vi "LIN speichern.vi"(8 "error in (no error)":errorcluster caption="Fehler (Eingang, kein Fehler)", 10 "File Name LIN":T2, 11 "Pfad LIN":T1) -> (0 "error out":errorcluster, 2 ".LIN Datei Pfad":path, 3 "Pfad LIN out":T1)   [LabVIEW 2020, in "Linearisierung v2.lvlib"]
uses:
  Linearisierung v2.lvlib
  Visualisierungs Elemente/Pfad-Eingabefeld.ctl
  Visualisierungs Elemente/String - Eingabefeld.ctl
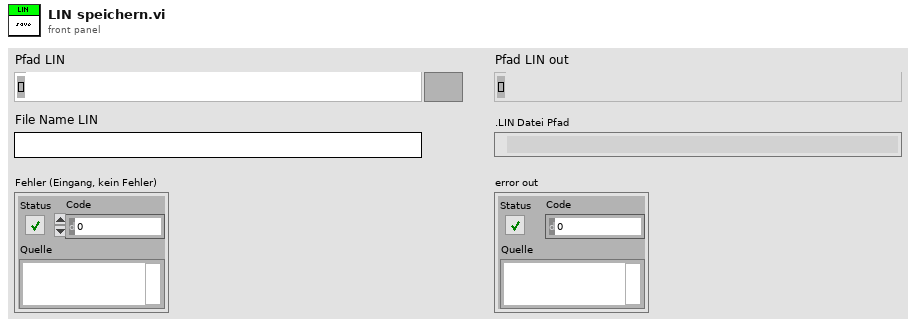
[diagram p1: front panel]
types:
  T1 = typedef "Pfad-Eingabefeld.ctl" = path
  T2 = typedef "String - Eingabefeld.ctl" = string
  T3 = enum16{"open", "replace", "create", "open or create", "replace or create", "replace or create with confirmation"}
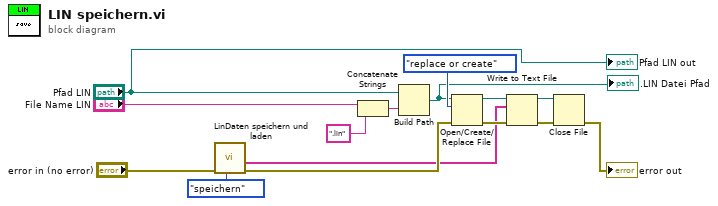
[diagram p0: block diagram]
diagram:
  n1 = call "LinDaten speichern und laden.vi"("Aktion"=enum16{"speichern", "laden"}."speichern", "error in (no error)"="error in (no error)") -> ("error out"=w4:errorcluster, "Daten zum Speichern"=w1:string[])  [unwired: 3 in, 5 out]
  n2 = Concatenate Strings("File Name LIN", ".lin" ("String")) -> (w5:string)
  n3 = Build Path(base path="Pfad LIN", name or relative path=w5) -> (appended path=w7:path)
  ".LIN Datei Pfad" <- w7
  n4 = Open/Create/Replace File(file path (use dialog)=w7, error in=w4, operation (0:open)=T3."replace or create" ("Operation (0:Öffnen)")) -> (refnum out=w10:refnum<file>, error out=w9:errorcluster)  [unwired: 3 in, 1 out]
  n5 = Write to Text File(file (use dialog)=w10, text=w1, error in=w9) -> (refnum out=w8:refnum<file>, error out=w14:errorcluster)  [unwired: 1 in, 1 out]
  n6 = Close File(refnum=w8, error in=w14) -> (error out=→"error out":errorcluster)  [unwired: 1 out]
  "Pfad LIN out" <- "Pfad LIN"
